vi "configure DAQ instrument.vi"(0 "Resource name":refnum<k15>="DAQ::1", 1 "Record length":i32=1000 caption="Min record length", 3 "Fetch number":i32, 4 "Trigger delay":dbl format="%.4f", 5 "Vertical range":dbl=10.0 format="%.2f", 6 "Trigger source":T1="0" caption="Trigger source (Channel 0)", 7 "Error in":errorcluster caption="error in", 9 "Channels":string="0", 11 "Sample rate":dbl=20000000.0 caption="Min sample rate", 12 "Number of records":i32=1, 13 "Trigger level":dbl format="%.2f") -> (10 "Instrument handle out":refnum<k15>, 15 "Error out":errorcluster caption="error out")   [LabVIEW 2014]
uses:
  <instrlib>/niScope/Controls/niScope trigger source.ctl
  <instrlib>/niScope/Controls/niScope trigger slope.ctl
  <instrlib>/niScope/Controls/niScope trigger coupling.ctl
  <instrlib>/niScope/Configure/Trigger/niScope Configure Trigger Edge.vi
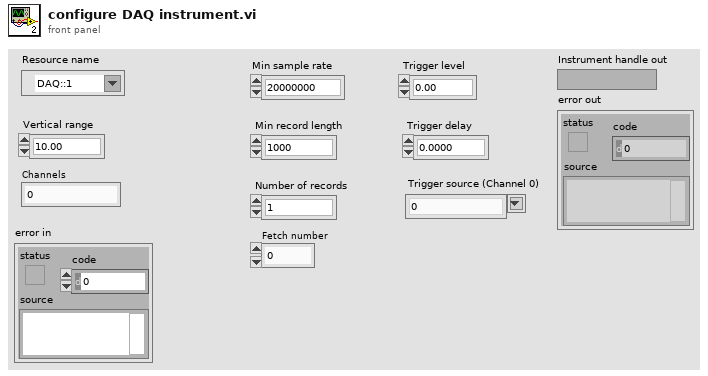
[diagram p1: front panel]
types:
  T1 = typedef "niScope trigger source.ctl" = string
  T2 = typedef "niScope trigger coupling.ctl" = u16
  T3 = typedef "niScope trigger slope.ctl" = i32
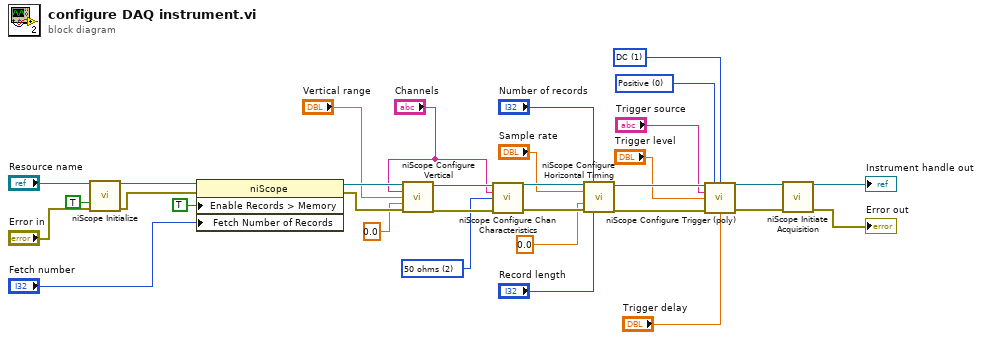
[diagram p0: block diagram]
diagram:
  w9 = T2 1 items=["AC"=0, "DC"=1, "HF Reject"=3, "LF Reject"=4, "AC Plus HF Reject"=1001] ("trigger coupling")
  w10 = T3 0 items=["Positive", "Negative"] ("trigger slope")
  w22 = u32 2 items=["1 mega ohm"=0, "50 ohms"=2] ("input impedance")
  n1 = call <instrlib>:"niScope Initialize.vi"("resource name"="Resource name", "reset device"=TRUE, "error in"="Error in") -> ("instrument handle"=w31:refnum<k15>, "error out"=w2:errorcluster)  [unwired: 11 in]
  n2 = property class="niScope"(reference=w31, error in=w2, "Enable Records > Memory"=TRUE ("Horizontal:Enable Records > Memory"), "Fetch Number of Records"="Fetch number") -> (reference out=w28:refnum<k15>, error out=w27:errorcluster)
  n3 = call <instrlib>:"niScope Configure Vertical.vi"("instrument handle"=w28, "channels"="Channels", "vertical range"="Vertical range", "vertical offset"=0.0, "error in"=w27) -> ("instrument handle out"=w24:refnum<k15>, "error out"=w23:errorcluster)  [unwired: 9 in]
  n4 = call <instrlib>:"niScope Configure Chan Characteristics.vi"("instrument handle"=w24, "channels"="Channels", "input impedance"=w22, "error in"=w23) -> ("instrument handle out"=w21:refnum<k15>, "error out"=w20:errorcluster)  [unwired: 10 in]
  n5 = call <instrlib>:"niScope Configure Horizontal Timing.vi"("instrument handle"=w21, "number of records"="Number of records", "min sample rate"="Sample rate", "reference position"=0.0, "error in"=w20, "min record length"="Record length") -> ("instrument handle out"=w15:refnum<k15>, "error out"=w14:errorcluster)  [unwired: 8 in]
  n6 = call-poly <instrlib>:"niScope Configure Trigger (poly).vi"("instrument handle"=w15, "trigger slope"=w10, "trigger coupling"=w9, "trigger source"="Trigger source", "trigger level"="Trigger level", "error in"=w14, "trigger delay"="Trigger delay") -> ("instrument handle out"=w8:refnum<k15>, "error out"=w7:errorcluster)  [unwired: 7 in]
  n7 = call <instrlib>:"niScope Initiate Acquisition.vi"("instrument handle"=w8, "error in"=w7) -> ("instrument handle out"=→"Instrument handle out":refnum<k15>, "error out"=→"Error out":errorcluster)  [unwired: 12 in]
